vi "Controller.vi"(10 "Sensors":T2) -> (0 "To Target Lossy Data":T1, 3 "Motor Command":dbl)   [LabVIEW 2018]
uses:
  Sensor Data.ctl
  Phase Calculator Feedback Cluster.ctl
  STTTM Cluster.ctl
  Target Lossy Data.ctl
panel:
  in  "Target Lossy Data":T1
  in  "STTTM - Thresholds, Parameters, and Previous Signal Value":T3
  in  "Phase Calculator Feedback":T4
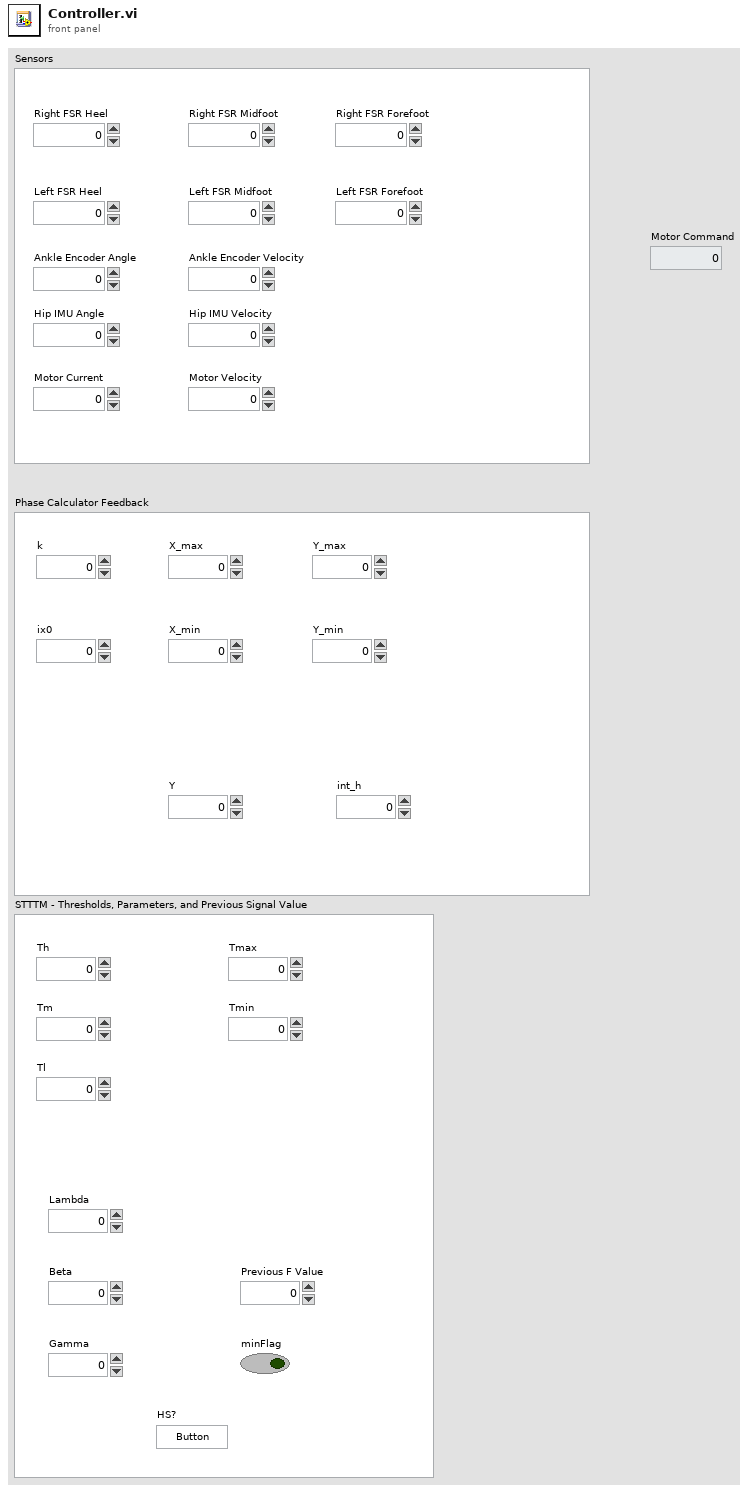
[diagram p1: front panel]
types:
  T1 = typedef "Target Lossy Data.ctl" = cluster{"Active Controller":bool, "Log Trigger":bool, "Sensors":T2, "Motor Command":dbl, "Phase Variable":dbl, "HS State":bool, "Heel Strike Pulse":bool, "Gait %":dbl, "Torque Reference":dbl, "Passive Torque":dbl, "High FSR Threshold":dbl, "Middle FSR Threshold":dbl, "Low FSR Threshold":dbl}
  T2 = typedef "Sensor Data.ctl" = cluster{"Motor Current":dbl, "Motor Velocity":dbl, "Hip IMU Angle":dbl, "Ankle Encoder Velocity":dbl, "Ankle Encoder Angle":dbl, "Hip IMU Velocity":dbl, "Left FSR Heel":dbl, "Left FSR Midfoot":dbl, "Left FSR Forefoot":dbl, "Right FSR Forefoot":dbl, "Right FSR Midfoot":dbl, "Right FSR Heel":dbl}
  T3 = typedef "STTTM Cluster.ctl" = cluster{"Th":dbl, "Tm":dbl, "Tl":dbl, "Tmax":dbl, "Tmin":dbl, "Lambda":dbl, "Beta":dbl, "Gamma":dbl, "Previous F Value":dbl, "minFlag":bool, "HS?":bool}
  T4 = typedef "Phase Calculator Feedback Cluster.ctl" = cluster{"k":dbl, "ix0":dbl, "X_max":dbl, "X_min":dbl, "Y_max":dbl, "Y_min":dbl, "Y":dbl, "int_h":dbl}
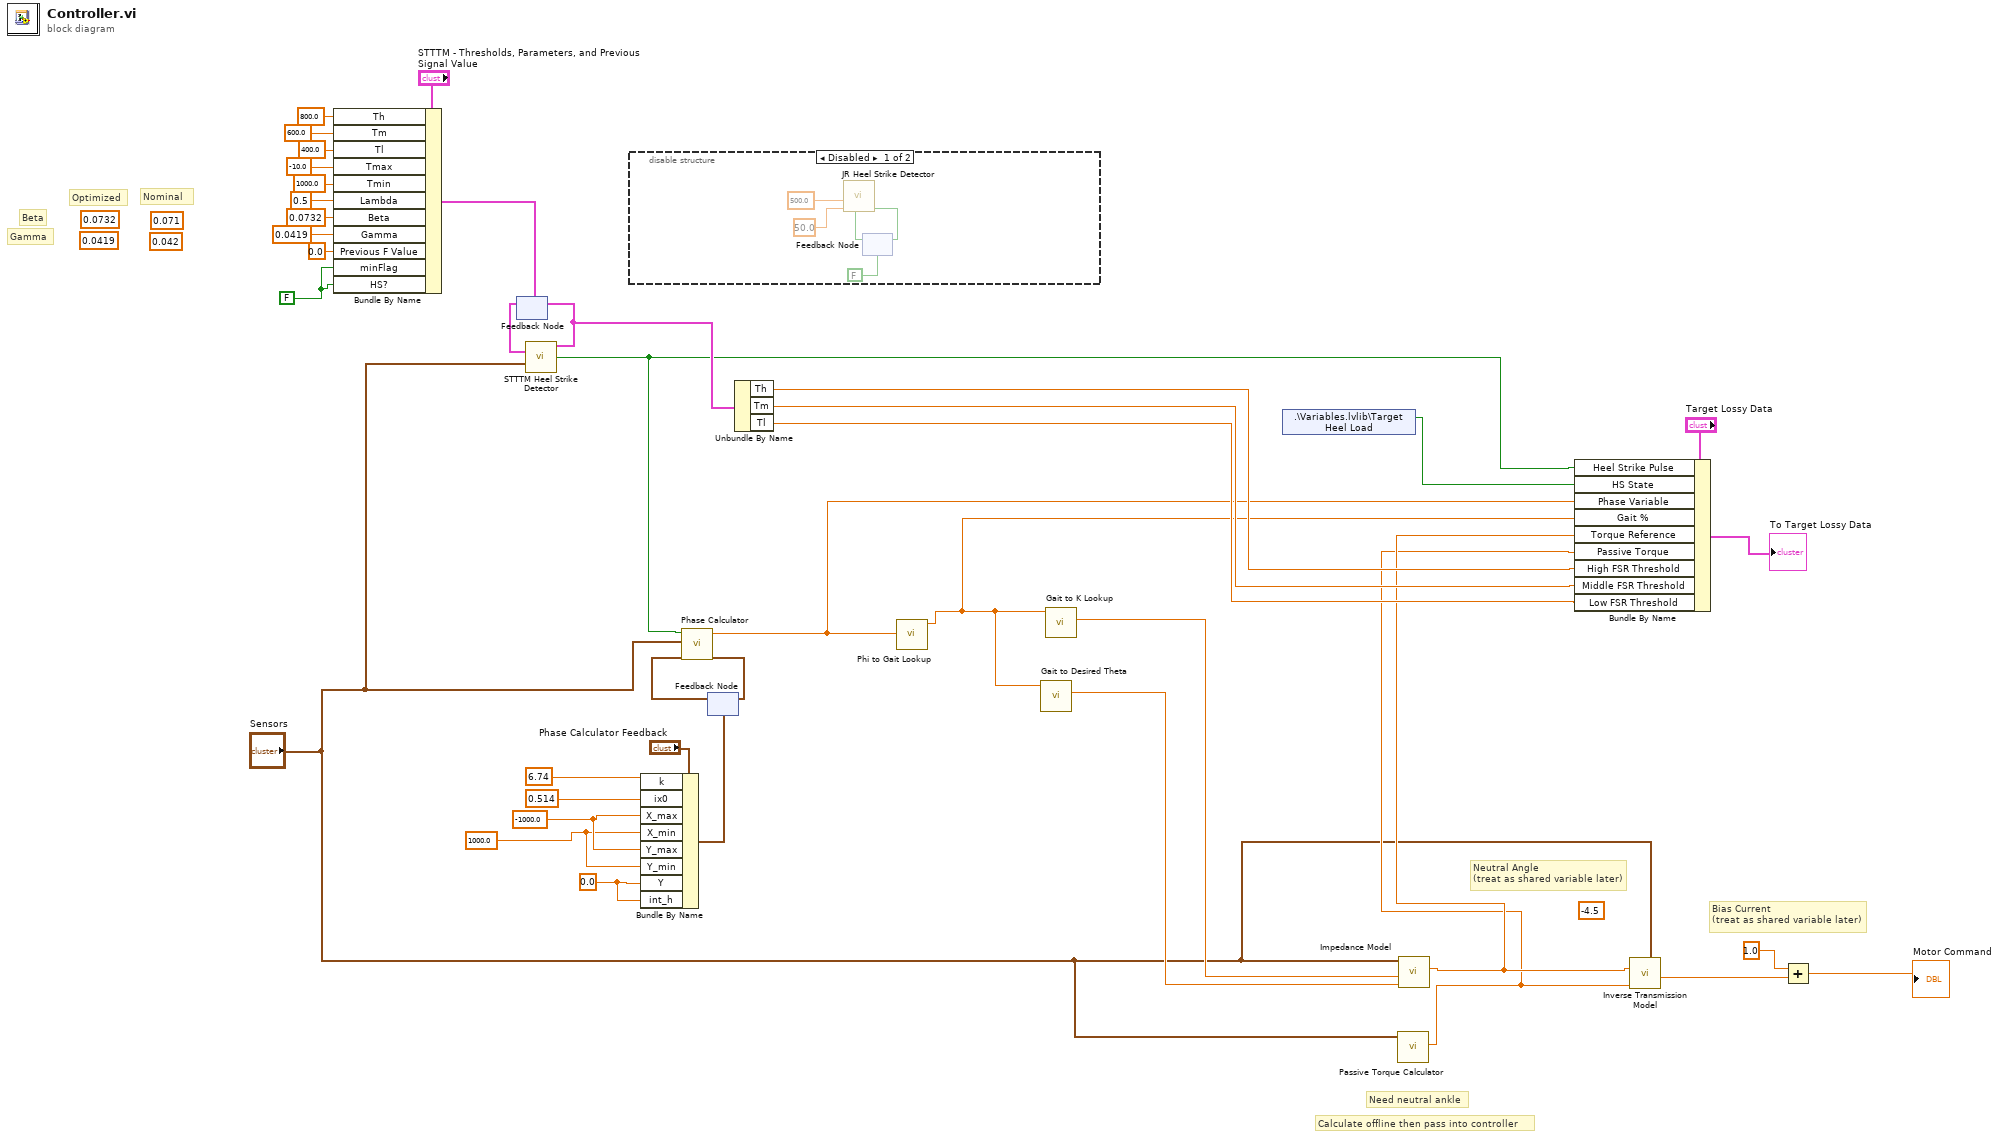
[diagram p0: block diagram]
diagram:
  (unwired) 0.042 ("Gamma")
  (unwired) 0.071 ("Beta")
  (unwired) 0.0419 ("Gamma")
  (unwired) 0.0732 ("Beta")
  w1 = FALSE ("minFlag")
  w30 = 0.0 ("Y")
  w33 = 1000.0 ("X_min")
  w34 = -1000.0 ("X_max")
  (unwired) -4.5
  # "Nominal"
  # "Gamma"
  # "Beta"
  # "Optimized"
  # "Bias Current \n(treat as shared variable later)"
  # "Neutral Angle \n(treat as shared variable later)"
  # "Calculate offline then pass into controller"
  # "Need neutral ankle"
  n1 = Bundle By Name(cluster="STTTM - Thresholds, Parameters, and Previous Signal Value", "Th"=800.0, "Tm"=600.0, "Tl"=400.0, "Tmax"=-10.0, "Tmin"=1000.0, "Lambda"=0.5, "Beta"=0.0732, "Gamma"=0.0419, "Previous F Value"=0.0, "minFlag"=w1, "HS?"=w1) -> (w28:T3)
  n2 = feedback #1(w28) -> (w29:T3)
  n3 = call "STTTM Heel Strike Detector.vi"("Sensors"="Sensors", "STTTM - Thresholds, Parameters, and Previous Signal Value (IN)"=w29) -> ("Heel Strike?"=w3:bool, "STTTM - Thresholds, Parameters, and Previous Signal Value (OUT)"=w16:T3)  [unwired: 7 in]
  n4 = feedback-in #1(w16) -> ()
  n5 = disable-structure shown="Disabled" {
    frame Disabled {
      n6 = feedback #2(FALSE) -> (w44:bool)
      n7 = call "JR Heel Strike Detector.vi"("Previous HS State"=w44, "Force Rate Threshold"=50.0, "Force Threshold"=500.0) -> ("Previous HS State"=w45:bool)  [unwired: 7 in, 1 out]
      n8 = feedback-in #2(w45) -> ()
    }
    frame Enabled {
    }
  }
  n9 = Bundle By Name(cluster="Phase Calculator Feedback", "k"=6.74, "ix0"=0.514, "X_max"=w34, "X_min"=w33, "Y_max"=w34, "Y_min"=w33, "Y"=w30, "int_h"=w30) -> (w37:T4)
  n10 = feedback #3(w37) -> (w31:T4)
  n11 = call "Phase Calculator.vi"("Feedback In"=w31, "Sensors"="Sensors", "Heel Strike?"=w3) -> ("Feedkback Out"=w32:T4, "Phase Angle (Phi)"=w9:dbl)  [unwired: 7 in]
  n12 = feedback-in #3(w32) -> ()
  n13 = Unbundle By Name(w16) -> ("Th"=w15:dbl, "Tm"=w14:dbl, "Tl"=w13:dbl)
  n14 = call "Phi to Gait Lookup.vi"("Current Phi"=w9) -> ("Current Gait %"=w12:dbl)  [unwired: 10 in]
  n15 = call "Gait to Desired Theta.vi"("Current Gait %"=w12) -> ("Current Desired Theta"=w39:dbl)  [unwired: 10 in]
  n16 = call "Gait to K Lookup.vi"("Current Gait %"=w12) -> ("Current K"=w40:dbl)  [unwired: 10 in]
  n17 = shared-variable ".\\Variables.lvlib\\Target Heel Load"() -> (w4:bool)  [unwired: 1 in, 1 out]
  n18 = call "Passive Torque Calculator.vi"("Sensors"="Sensors") -> ("Passive Torque Estimate"=w10:dbl)  [unwired: 10 in]
  n19 = call "Impedance Model.vi"("Theta_d"=w39, "K"=w40, "Sensors"="Sensors") -> ("Tau_ref"=w11:dbl)  [unwired: 8 in]
  n20 = Bundle By Name(cluster="Target Lossy Data", "Heel Strike Pulse"=w3, "HS State"=w4, "Phase Variable"=w9, "Gait %"=w12, "Torque Reference"=w11, "Passive Torque"=w10, "High FSR Threshold"=w15, "Middle FSR Threshold"=w14, "Low FSR Threshold"=w13) -> (→"To Target Lossy Data":T1)
  n21 = call "Inverse Transmission Model.vi"("Sensors"="Sensors", "Passive Torque Estimate"=w10, "Torque Reference"=w11) -> ("Motor Command"=w7:dbl)  [unwired: 8 in]
  n22 = Add(x=1.0, y=w7) -> (x+y=→"Motor Command":dbl)
